vi "Cut Spectrum FWHM.vi"(2 "XScale.Maximum":dbl format="%.2f", 3 "XScale.Minimum":dbl format="%.2f", 4 "Intensities":dbl[](array[numeric]) format="%.2f", 5 "Wavelengths":dbl[](array[numeric]) format="%.2f") -> (0 "Cut Intensities":dbl[](array[numeric]) format="%.2f", 1 "FWHM":dbl format="%.2f")   [LabVIEW 2023]
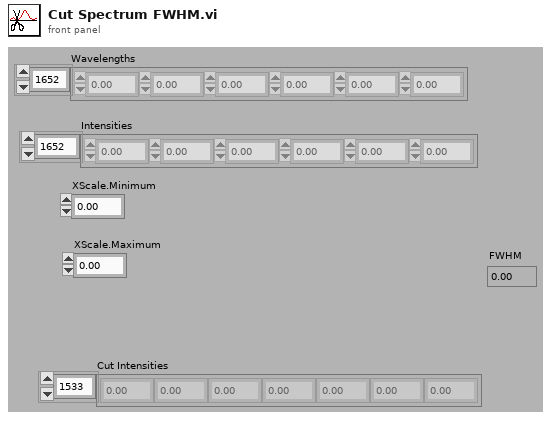
[diagram p1: front panel]
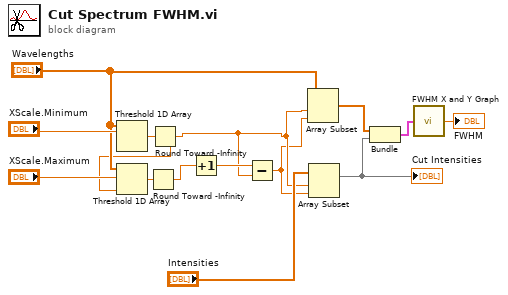
[diagram p0: block diagram]
diagram:
  n1 = Threshold 1D Array(2:"XScale.Minimum", 3:"Wavelengths") -> (0:w13:dbl)  [unwired: 1 in]
  n2 = Round Toward -Infinity(1:w13) -> (0:w6:dbl)
  n3 = Threshold 1D Array(1:w6, 2:"XScale.Maximum", 3:"Wavelengths") -> (0:w14:dbl)
  n4 = Round Toward -Infinity(1:w14) -> (0:w9:dbl)
  n5 = Increment(x=w9) -> (x+1=w8:dbl)
  n6 = Subtract(x=w8, y=w6) -> (x-y=w5:dbl)
  n7 = Array Subset(array="Wavelengths", index=w6, length=w5) -> (w4:dbl[])
  n8 = Array Subset(array="Intensities", index=w6, length=w5) -> (w3:dbl[])
  "Cut Intensities" <- w3
  n9 = Bundle(w4, w3) -> (w2:cluster{dbl[], dbl[]})  [unwired: 1 in]
  n10 = call "FWHM X and Y Graph.vi"("Input Arrays"=w2) -> ("FWHM"=→"FWHM":dbl)
